vi "HumanProcessDPad.vi"(11 "POV":i16[](array[numeric])) -> (0 "Left":bool, 1 "Down":bool, 2 "Right":bool, 3 "Up":bool)   [LabVIEW 2023]
doc: "Process's the POV value of the Dpad into simple boolean outputs."
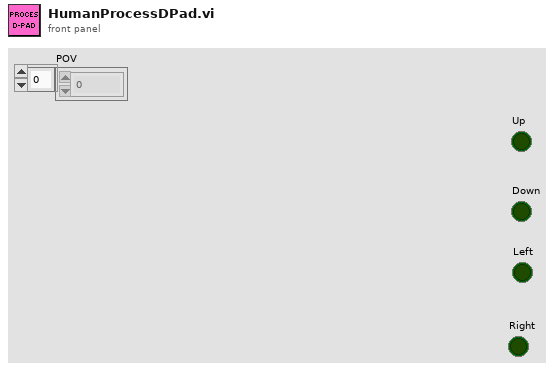
[diagram p1: front panel]
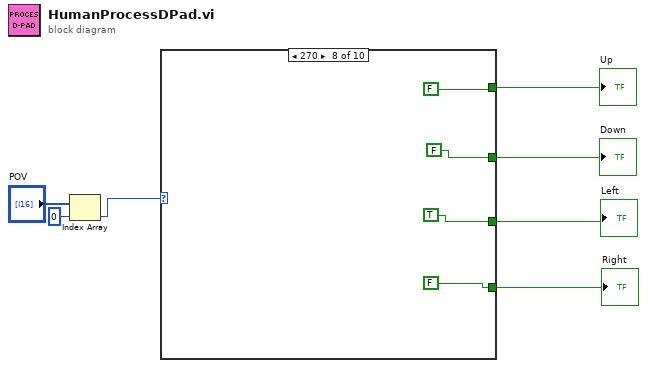
[diagram p0: block diagram]
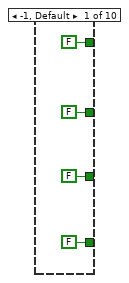
[diagram p2: hidden frame]
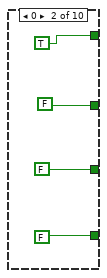
[diagram p3: hidden frame]
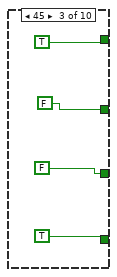
[diagram p4: hidden frame]
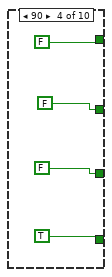
[diagram p5: hidden frame]
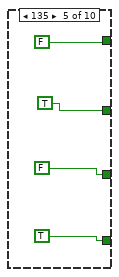
[diagram p6: hidden frame]
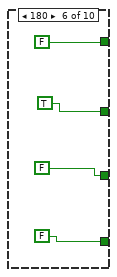
[diagram p7: hidden frame]
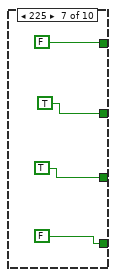
[diagram p8: hidden frame]
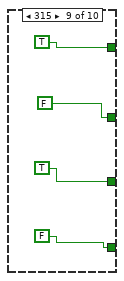
[diagram p9: hidden frame]
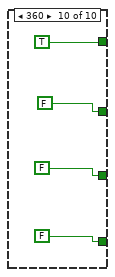
[diagram p10: hidden frame]
diagram:
  n1 = Index Array(array="POV", index=0) -> (element=w2:i16)
  n2 = case shown="270" w2 {
    tunnel: [FALSE TRUE TRUE FALSE FALSE FALSE FALSE FALSE TRUE TRUE] -> w7
    tunnel: [FALSE FALSE FALSE FALSE TRUE TRUE TRUE FALSE FALSE FALSE] -> w6
    tunnel: [FALSE FALSE FALSE FALSE FALSE FALSE TRUE TRUE TRUE FALSE] -> w5
    tunnel: [FALSE FALSE TRUE TRUE TRUE FALSE FALSE FALSE FALSE FALSE] -> w4
    frame -1, Default {
    }
    frame 0 {
    }
    frame 45 {
    }
    frame 90 {
    }
    frame 135 {
    }
    frame 180 {
    }
    frame 225 {
    }
    frame 270 {
    }
    frame 315 {
    }
    frame 360 {
    }
  }
  "Up" <- w7
  "Down" <- w6
  "Left" <- w5
  "Right" <- w4
